vi "ExampleGratingsWavelength.vi"() -> ()   [LabVIEW 2009]
uses:
  atspectrograph.lvlib
  C/Program Files (x86)/National Instruments/LabVIEW 2018/user.lib/ATSpectrograph/ATSpectrograph.llb/atspectrograph_portPosition_typedef.ctl
panel:
  in  "Device":i32 min=0 max=0
  in  "Set Device":bool
  in  "Tab Control":enum32{"GRATINGS", "WAVELENGTH"}(tab)
  in  "Exit Port":T1
  in  "Entrance Port":T1
  in  "Grating Offset":i32
  out "SetGratingOffset":string
  in  "Detector Offset":i32
  out "SetDetectorOffset":string
  out "WavelengthReset":string
  out "SetGrating":string
  in  "Grating":i32
  in  "Turret":i32
  out "SetTurret":string
  in  "SetGratingOffset":bool
  in  "SetDetectorOffset":bool
  in  "WavelengthReset":bool
  in  "SetGrating":bool
  in  "SetTurret":bool
  out "blaze":string
  out "Grating Offset":i32
  out "Detector Offset":i32
  out "offset":i32
  out "home":i32
  out "lines/mm":dbl format="%.2f"
  out "Grating":i32
  out "No Gratings":i32
  out "Turret":i32
  out "Is Grating ?":string
  out "GetGratingOffset":string
  out "GetDetectorOffset":string
  out "GetGratingInfo":string
  out "GetGrating":string
  out "GetNumberGratings":string
  out "GetTurret":string
  out "GratingIsPresent":string
  out "GotoZeroOrder":string
  out "SetWavelength":string
  in  "Wavelength":dbl format="%.2f"
  in  "GoToZeroOrder":bool
  out "Max Wavelength":dbl format="%.2f"
  out "Min Wavelength":dbl format="%.2f"
  out "Is Wavelength ?":string
  out "WavelengthIsPresent":string
  out "GetWavelengthLimits":string
  out "At Zero Order ?":string
  out "AtZeroOrder":string
  out "Wavelength":dbl format="%.2f"
  in  "SetWavelength 2":bool
  out "GetWavelength":string
  out "Initializing":bool
  in  "STOP if TRUE":bool
  out "Focal tilt":dbl format="%.2f"
  out "Angular Deviation":dbl format="%.2f"
  out "Focal length":dbl format="%.2f"
  out "Serial Number":string
  out "No of devices":i32
  out "GetOpticalParameters":string
  out "GetSerialNumber":string
  out "GetNumberDevices":string
  out "Close":string
  out "Initialize":string
  # "INITIALIZATION"
  # "SDK RETURN VALUES"
  # "SHAMROCK PARAMETERS"
  # "ACTIONS"
  # "SDK RETURN VALUES"
  # "SHAMROCK PARAMETERS"
  # "ACTIONS"
  # "SDK RETURN VALUES"
  # "SHAMROCK PARAMETERS"
  # "ACTIONS"
  # "nm"
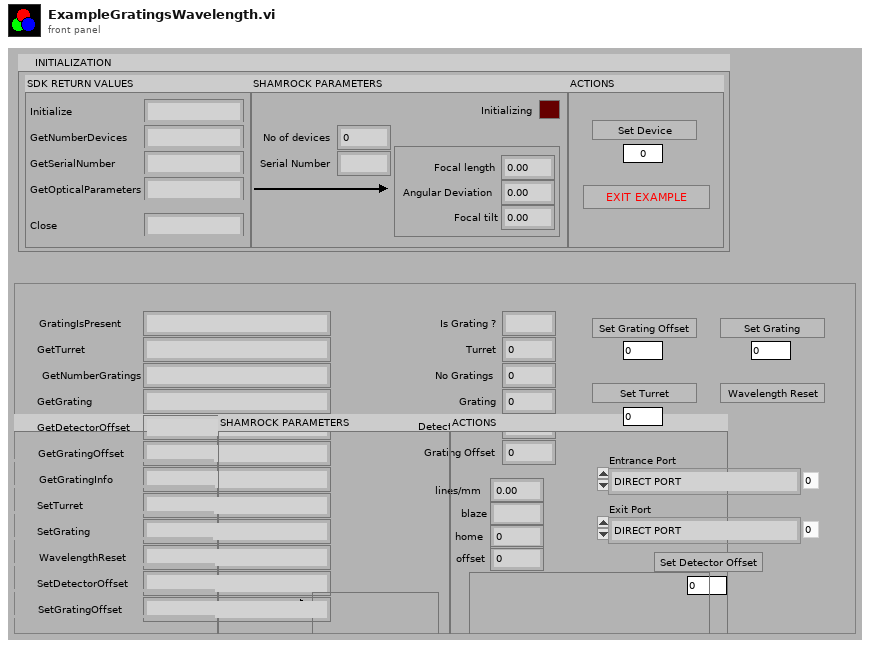
[diagram p1: front panel]
types:
  T1 = typedef "atspectrograph_portPosition_typedef.ctl" = enum32{"DIRECT PORT", "SIDE PORT"}
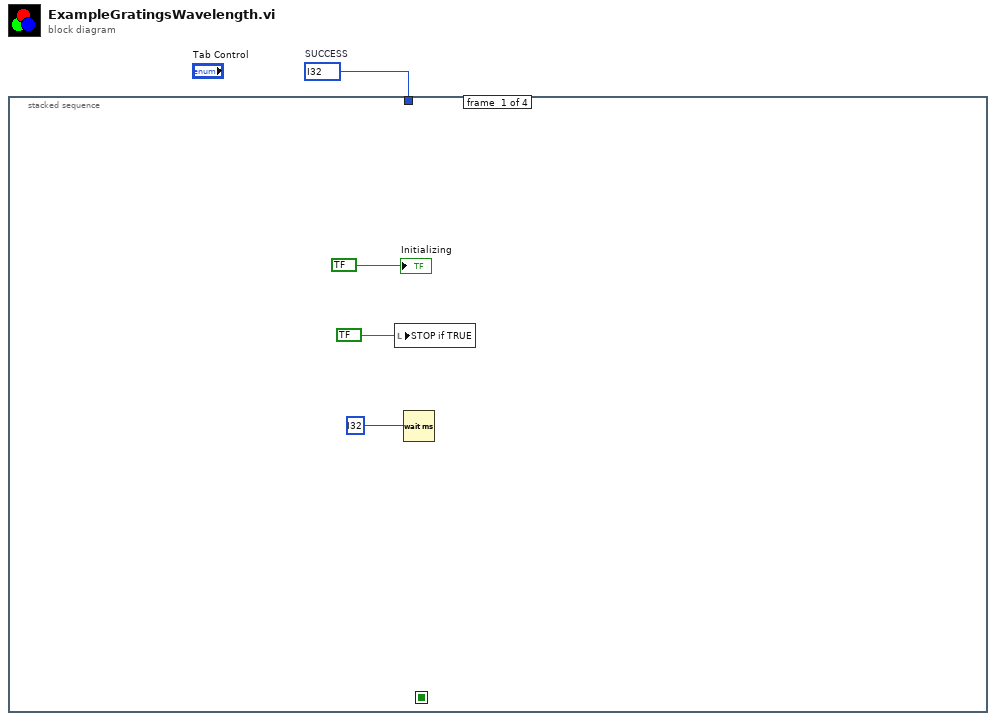
[diagram p0: block diagram]
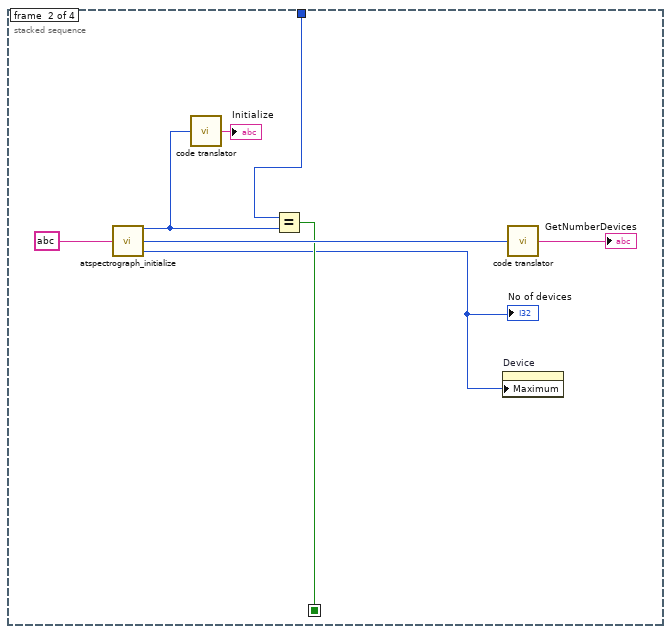
[diagram p2: hidden frame]
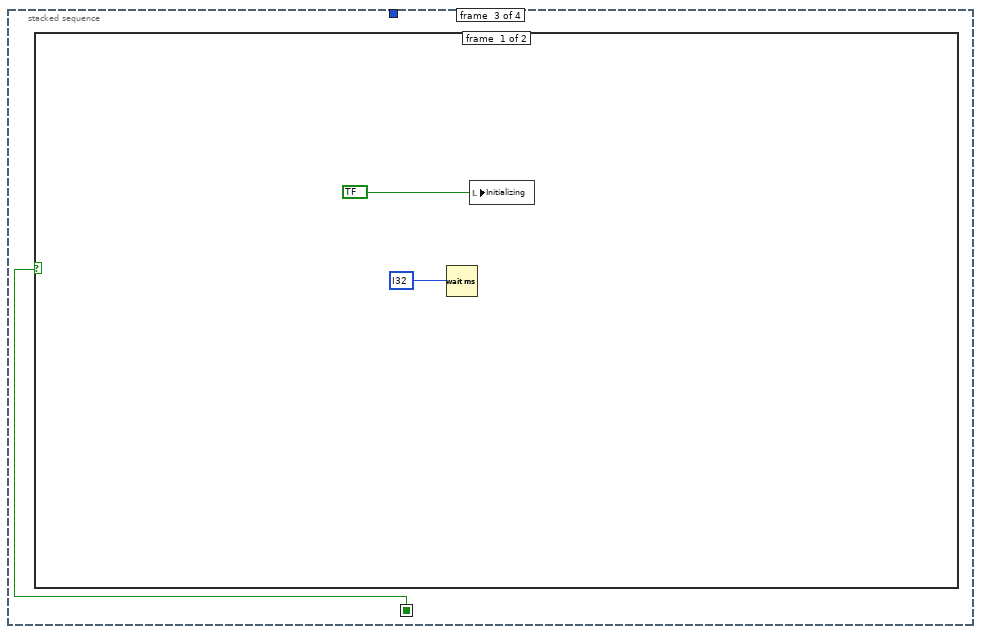
[diagram p3: hidden frame]
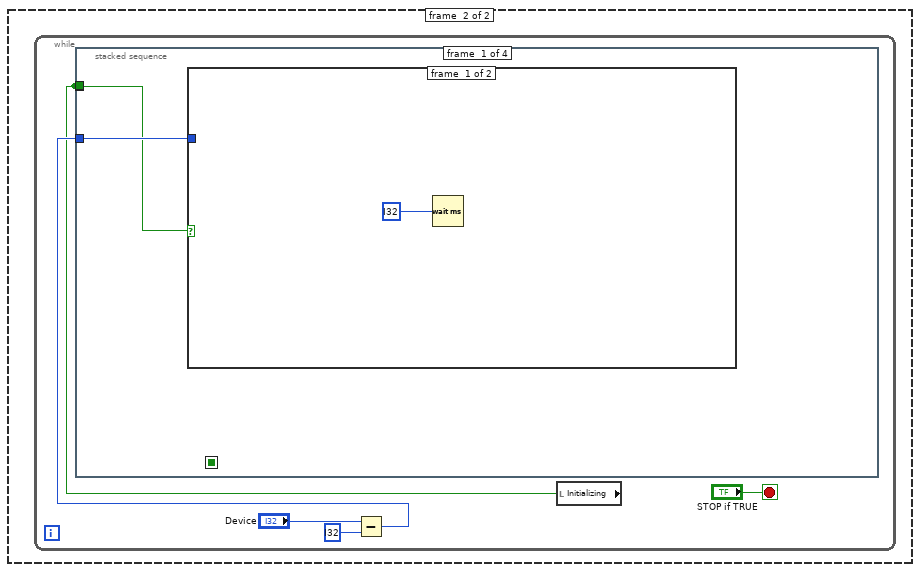
[diagram p4: hidden frame]
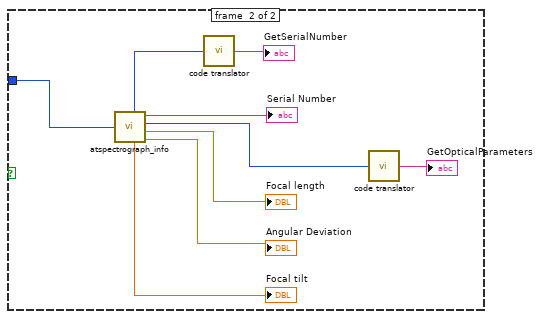
[diagram p5: hidden frame]
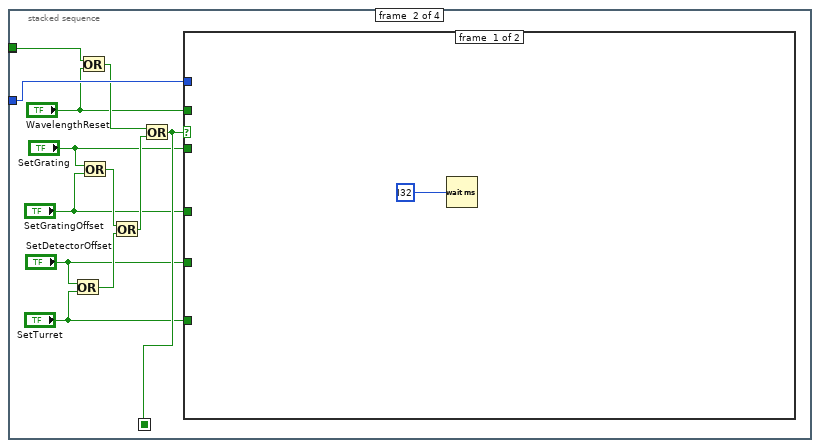
[diagram p6: hidden frame]
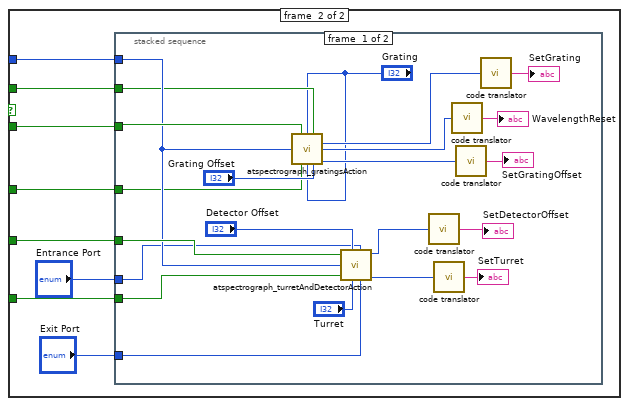
[diagram p7: hidden frame]
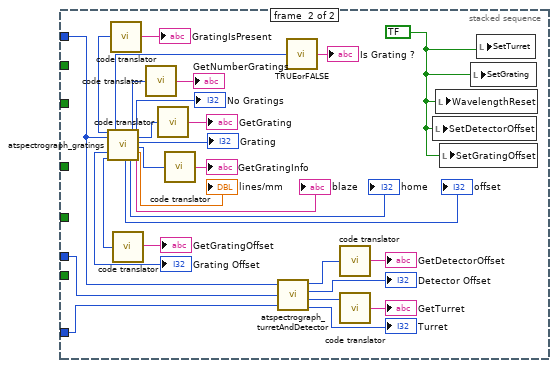
[diagram p8: hidden frame]
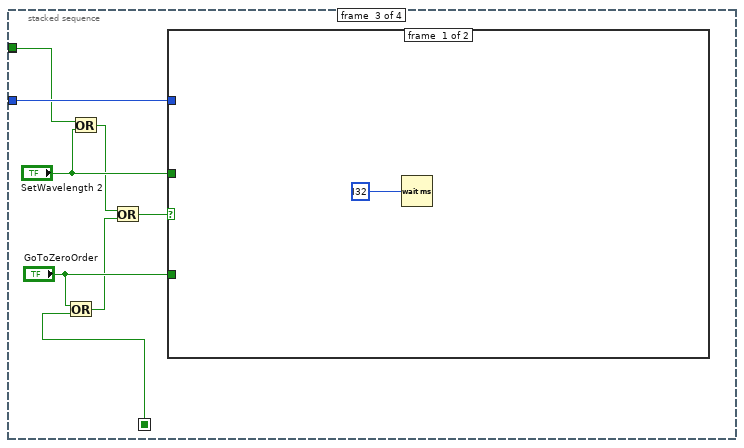
[diagram p9: hidden frame]
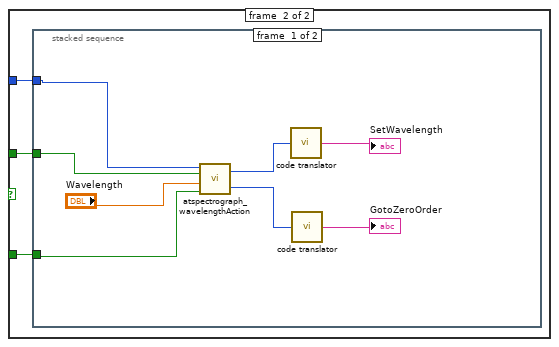
[diagram p10: hidden frame]
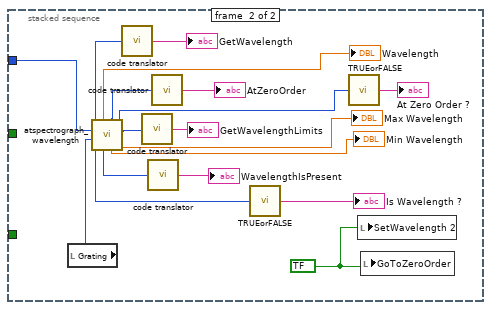
[diagram p11: hidden frame]
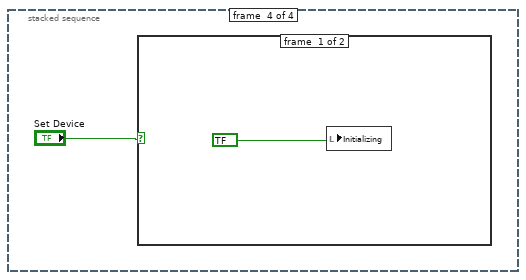
[diagram p12: hidden frame]
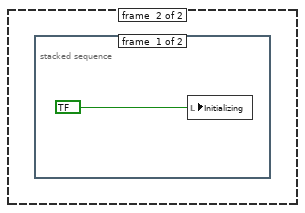
[diagram p13: hidden frame]
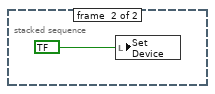
[diagram p14: hidden frame]
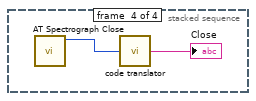
[diagram p15: hidden frame]
diagram:
  w1 = i32 ?  # SUCCESS
  n1 = stacked-sequence {
    seq-local: [_ w6 _ _] -> [_ _ w13 _]
    tunnel: w1 -> [_ w12 _ _]
    frame #0 {
      n2 = local write "STOP if TRUE"(bool ?) -> ()
      n3 = Wait (ms)(milliseconds to wait=i32 ?) -> ()  [unwired: 1 out]
      "Initializing" <- bool ?
    }
    frame #1 {
      n4 = call "atspectrograph_initialize.vi"("Initialization path"=string ?) -> ("RC_Initialize"=w9:u32, "RC_GetNumberDevices"=w8:u32, "No Devices"=w5:i32)
      "No of devices" <- w5
      n5 = call "code translator.vi"("Error code"=w9) -> ("Error description"=→"Initialize":string)
      n6 = Equal?(x=w12, y=w9) -> (x = y?=w6:bool)
      n7 = property on="Device" class="DigNum (strict)"("Maximum"=w5) -> ()  [unwired: 2 in, 2 out]
      n8 = call "code translator.vi"("Error code"=w8) -> ("Error description"=→"GetNumberDevices":string)
    }
    frame #2 {
      n9 = case shown="True" w13 {
        frame #0 {
          n10 = Wait (ms)(milliseconds to wait=i32 ?) -> ()  [unwired: 1 out]
          n11 = local write "Initializing"(bool ?) -> ()
        }
        frame #1 {
          n12 = while {
            stop <- "STOP if TRUE" stop-if-true
            n13 = Subtract(x="Device", y=i32 ?) -> (x-y=w19:i32)
            n14 = local read "Initializing"() -> (w16:bool)
            n15 = stacked-sequence {
              seq-local: [_ w38 _ _] -> [_ _ w111 _]
              tunnel: w19 -> [w22 w44 w112 _]
              tunnel: w16 -> [w21 w41 w108 _]
              tunnel: w16 -> [_ _ _ _]
              frame #0 {
                n16 = case shown="True" w21 {
                  tunnel: w22 -> [_ w24]
                  frame #0 {
                    n17 = Wait (ms)(milliseconds to wait=i32 ?) -> ()  [unwired: 1 out]
                  }
                  frame #1 {
                    n18 = call "atspectrograph_info.vi"("Device No"=w24) -> ("RC_GetSerialNumber"=w28:u32, "Focal Tilt"=→"Focal tilt":sgl, "Serial Number"=→"Serial Number":string, "RC_GetOpticalParameters"=w26:u32, "Focal Length"=→"Focal length":sgl, "Angular Deviation"=→"Angular Deviation":sgl)
                    n19 = call "code translator.vi"("Error code"=w28) -> ("Error description"=→"GetSerialNumber":string)
                    n20 = call "code translator.vi"("Error code"=w26) -> ("Error description"=→"GetOpticalParameters":string)
                  }
                }
              }
              frame #1 {
                n21 = Or(x="SetDetectorOffset", y="SetTurret") -> (x .or. y?=w42:bool)
                n22 = Or(x=w41, y="WavelengthReset") -> (x .or. y?=w40:bool)
                n23 = Or(x="SetGrating", y="SetGratingOffset") -> (x .or. y?=w43:bool)
                n24 = Or(x=w43, y=w42) -> (x .or. y?=w39:bool)
                n25 = Or(x=w40, y=w39) -> (x .or. y?=w38:bool)
                n26 = case shown="True" w38 {
                  tunnel: w44 -> [_ w53]
                  tunnel: "SetDetectorOffset" -> [_ w52]
                  tunnel: "SetTurret" -> [_ w51]
                  tunnel: "SetGrating" -> [_ w50]
                  tunnel: "SetGratingOffset" -> [_ w49]
                  tunnel: "WavelengthReset" -> [_ w48]
                  frame #0 {
                    n27 = Wait (ms)(milliseconds to wait=i32 ?) -> ()  [unwired: 1 out]
                  }
                  frame #1 {
                    n28 = stacked-sequence {
                      tunnel: w48 -> [w59 _]
                      tunnel: w53 -> [w62 w82]
                      tunnel: w50 -> [w74 _]
                      tunnel: w49 -> [w57 _]
                      tunnel: w52 -> [w63 _]
                      tunnel: w51 -> [w56 _]
                      tunnel: "Entrance Port" -> [w55 w77]
                      tunnel: "Exit Port" -> [w54 w76]
                      frame #0 {
                        n29 = call "atspectrograph_gratingsAction.vi"("WavelengthReset"=w59, "Grating Offset"="Grating Offset", 7:"Grating"="Grating", 8:"Grating"="Grating", "SetGrating"=w74, "SetGratingOffset"=w57, "Device No"=w62) -> ("RC_SetGrating"=w72:u32, "RC_WavelengthReset"=w69:u32, "RC_SetGratingOffset"=w67:u32)  [unwired: 6 in]
                        n30 = call "atspectrograph_turretAndDetectorAction.vi"("SetDetectorOffset"=w63, "Detector Offset"="Detector Offset", "Device No"=w62, "SetTurret"=w56, "Turret"="Turret", "Entrance Port"=w55, "Exit Port"=w54) -> ("RC_SetDetectorOffset"=w61:u32, "RC_SetTurret"=w60:u32)  [unwired: 2 in]
                        n31 = call "code translator.vi"("Error code"=w61) -> ("Error description"=→"SetDetectorOffset":string)
                        n32 = call "code translator.vi"("Error code"=w60) -> ("Error description"=→"SetTurret":string)
                        n33 = call "code translator.vi"("Error code"=w69) -> ("Error description"=→"WavelengthReset":string)
                        n34 = call "code translator.vi"("Error code"=w67) -> ("Error description"=→"SetGratingOffset":string)
                        n35 = call "code translator.vi"("Error code"=w72) -> ("Error description"=→"SetGrating":string)
                      }
                      frame #1 {
                        w104 = bool ?
                        n36 = call "atspectrograph_gratings.vi"("Device No"=w82) -> ("No Gratings"=→"No Gratings":i32, "RC_GetNumberGratings"=w93:u32, "Is Present"=w84:i32, "RC_GratingIsPresent"=w96:u32, "RC_GetGrating"=w91:u32, "Grating"=→"Grating":i32, "RC_GetGratingInfo"=w89:u32, "Lines/mm"=→"lines/mm":sgl, "Grating Offset"=→"Grating Offset":i32, "Blaze"=→"blaze":string, "Home"=→"home":i32, "Offset"=→"offset":i32, "RC_GetGratingOffset"=w86:u32)  [unwired: 6 in]
                        n37 = call "code translator.vi"("Error code"=w96) -> ("Error description"=→"GratingIsPresent":string)
                        n38 = call "code translator.vi"("Error code"=w86) -> ("Error description"=→"GetGratingOffset":string)
                        n39 = call "code translator.vi"("Error code"=w93) -> ("Error description"=→"GetNumberGratings":string)
                        n40 = call "code translator.vi"("Error code"=w91) -> ("Error description"=→"GetGrating":string)
                        n41 = call "code translator.vi"("Error code"=w89) -> ("Error description"=→"GetGratingInfo":string)
                        n42 = call "atspectrograph_turretAndDetector.vi"("Device No"=w82, "Entrance Port"=w77, "Exit Port"=w76) -> ("RC_GetDetectorOffset"=w79:u32, "Detector Offset"=→"Detector Offset":i32, "RC_GetTurret"=w81:u32, "Turret"=→"Turret":i32)
                        n43 = call "TRUEorFALSE.vi"("bool number"=w84) -> ("String"=→"Is Grating ?":string)
                        n44 = call "code translator.vi"("Error code"=w79) -> ("Error description"=→"GetDetectorOffset":string)
                        n45 = call "code translator.vi"("Error code"=w81) -> ("Error description"=→"GetTurret":string)
                        n46 = local write "SetDetectorOffset"(w104) -> ()
                        n47 = local write "WavelengthReset"(w104) -> ()
                        n48 = local write "SetGratingOffset"(w104) -> ()
                        n49 = local write "SetGrating"(w104) -> ()
                        n50 = local write "SetTurret"(w104) -> ()
                      }
                    }
                  }
                }
              }
              frame #2 {
                n51 = Or(x="GoToZeroOrder", y=w111) -> (x .or. y?=w106:bool)
                n52 = Or(x=w108, y="SetWavelength 2") -> (x .or. y?=w107:bool)
                n53 = Or(x=w107, y=w106) -> (x .or. y?=w105:bool)
                n54 = case shown="True" w105 {
                  tunnel: "SetWavelength 2" -> [_ w116]
                  tunnel: "GoToZeroOrder" -> [_ w115]
                  tunnel: w112 -> [_ w114]
                  frame #0 {
                    n55 = Wait (ms)(milliseconds to wait=i32 ?) -> ()  [unwired: 1 out]
                  }
                  frame #1 {
                    n56 = stacked-sequence {
                      tunnel: w116 -> [w122 _]
                      tunnel: w115 -> [w123 _]
                      tunnel: w114 -> [w121 w137]
                      frame #0 {
                        n57 = call "atspectrograph_wavelengthAction.vi"("GoToZeroOrder"=w123, "Wavelength"="Wavelength", "SetWavelength"=w122, "Device No"=w121) -> ("RC_GotoZeroOrder"=w118:u32, "RC_SetWavelength"=w120:u32)
                        n58 = call "code translator.vi"("Error code"=w120) -> ("Error description"=→"SetWavelength":string)
                        n59 = call "code translator.vi"("Error code"=w118) -> ("Error description"=→"GotoZeroOrder":string)
                      }
                      frame #1 {
                        w142 = bool ?
                        n60 = local read "Grating"() -> (w138:i32)
                        n61 = call "atspectrograph_wavelength.vi"("Grating No"=w138, "Device No"=w137) -> ("Is Present"=w126:i32, "RC_WavelengthIsPresent"=w130:u32, "Min Wavelength"=→"Min Wavelength":sgl, "Max Wavelength"=→"Max Wavelength":sgl, "RC_GetWavelengthLimits"=w132:u32, "RC_GetWavelength"=w136:u32, "Wavelength"=→"Wavelength":sgl, "RC_AtZeroOrder"=w134:u32, "At Zero Order"=w128:i32)
                        n62 = call "code translator.vi"("Error code"=w136) -> ("Error description"=→"GetWavelength":string)
                        n63 = call "code translator.vi"("Error code"=w132) -> ("Error description"=→"GetWavelengthLimits":string)
                        n64 = call "code translator.vi"("Error code"=w130) -> ("Error description"=→"WavelengthIsPresent":string)
                        n65 = call "code translator.vi"("Error code"=w134) -> ("Error description"=→"AtZeroOrder":string)
                        n66 = call "TRUEorFALSE.vi"("bool number"=w126) -> ("String"=→"Is Wavelength ?":string)
                        n67 = call "TRUEorFALSE.vi"("bool number"=w128) -> ("String"=→"At Zero Order ?":string)
                        n68 = local write "SetWavelength 2"(w142) -> ()
                        n69 = local write "GoToZeroOrder"(w142) -> ()
                      }
                    }
                  }
                }
              }
              frame #3 {
                n70 = case shown="True" "Set Device" {
                  frame #0 {
                    n71 = local write "Initializing"(bool ?) -> ()
                  }
                  frame #1 {
                    n72 = stacked-sequence {
                      frame #0 {
                        n73 = local write "Initializing"(bool ?) -> ()
                      }
                      frame #1 {
                        n74 = local write "Set Device"(bool ?) -> ()
                      }
                    }
                  }
                }
              }
            }
          }
        }
      }
    }
    frame #3 {
      n75 = call "AT Spectrograph Close.vi"() -> ("function return"=w148:u32)  [unwired: 11 in]
      n76 = call "code translator.vi"("Error code"=w148) -> ("Error description"=→"Close":string)
    }
  }
